vi "Nitro and Dut.vi"(11 "Stand in":refnum<class "Stand.lvclass">) -> (3 "nitro and dut":bool)   [LabVIEW 2019, in "Stand.lvclass"]
uses:
  Stand.lvclass
  Stand.lvclass/Stand.ctl
  TypeDef/Direction.ctl
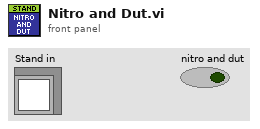
[diagram p1: front panel]
types:
  T1 = typedef "Direction.ctl" = enum8{"DUT", "Chamber"}
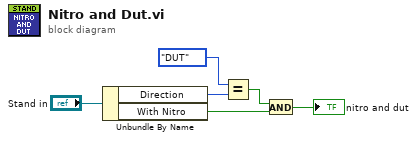
[diagram p0: block diagram]
diagram:
  n1 = Unbundle By Name("Stand in") -> ("Direction"=w1:T1, "With Nitro"=w4:bool)
  n2 = Equal?(x=Direction."DUT", y=w1) -> (x = y?=w5:bool)
  n3 = And(x=w5, y=w4) -> (x .and. y?=→"nitro and dut":bool)
